vi "_Write.vi"(8 "error in (no error)":errorcluster, 9 "Timeout S (0)":dbl, 10 "Data":string, 11 "DeployTCPResource in":refnum<class "TCPResource.lvclass">) -> (0 "error out":errorcluster, 2 "Bytes Written":i32, 3 "DeployTCPResource out":refnum<class "TCPResource.lvclass">)   [LabVIEW 2020, in "PicoG-Core.lvlib" / "TCPResource.lvclass"]
uses:
  TCPResource.lvclass
  TCPResource.lvclass/TCPResource.ctl
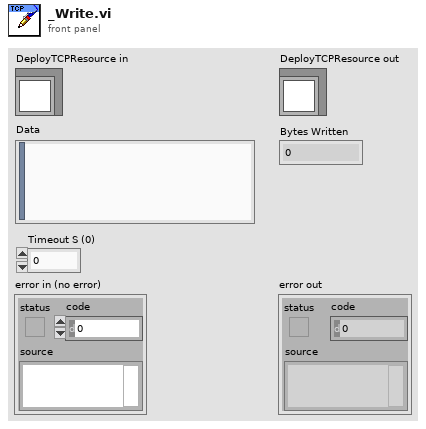
[diagram p1: front panel]
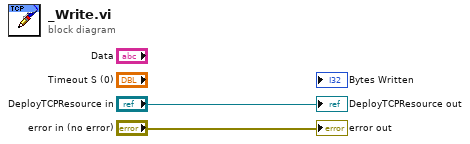
[diagram p0: block diagram]
diagram:
  "error out" <- "error in (no error)"
  "DeployTCPResource out" <- "DeployTCPResource in"
